vi "Store Packet.vi"(8 "error in (no error)":errorcluster, 9 "last attempt (now)":timestamp, 10 "ControlPacket":refnum<class "ControlPacket.lvclass">, 11 "Subscription in":refnum<class "Subscription.lvclass">) -> (0 "error out":errorcluster, 2 "ControlPacket dup":refnum<class "ControlPacket.lvclass">, 3 "Subscription out":refnum<class "Subscription.lvclass">)   [LabVIEW 2013, in "MQTT Server.lvlib" / "Subscription.lvclass"]
uses:
  Subscription.lvclass
  <vilib>/LabVIEW Open Source Project/MQTT Control Packets/Control Packets/ControlPacket/ControlPacket.lvclass
  Stored Packet -- cluster.ctl
  Subscription.lvclass/Subscription.ctl
  <vilib>/LabVIEW Open Source Project/MQTT Control Packets/Control Packets/ControlPacket/ControlPacket.lvclass/ControlPacket.ctl
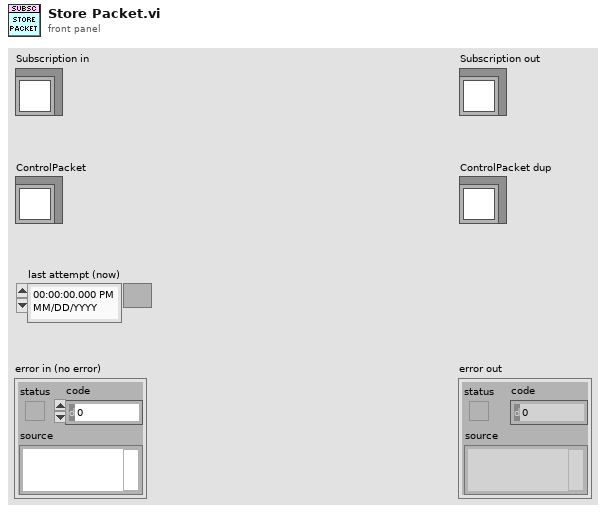
[diagram p1: front panel]
types:
  T1 = typedef "MQTT Server.lvlib/Subscription.lvclass/Stored Packet -- cluster.ctl" = cluster{"Packet Identifier":u16, "ControlPacket":refnum<class "ControlPacket.lvclass">, "last attempt":timestamp}
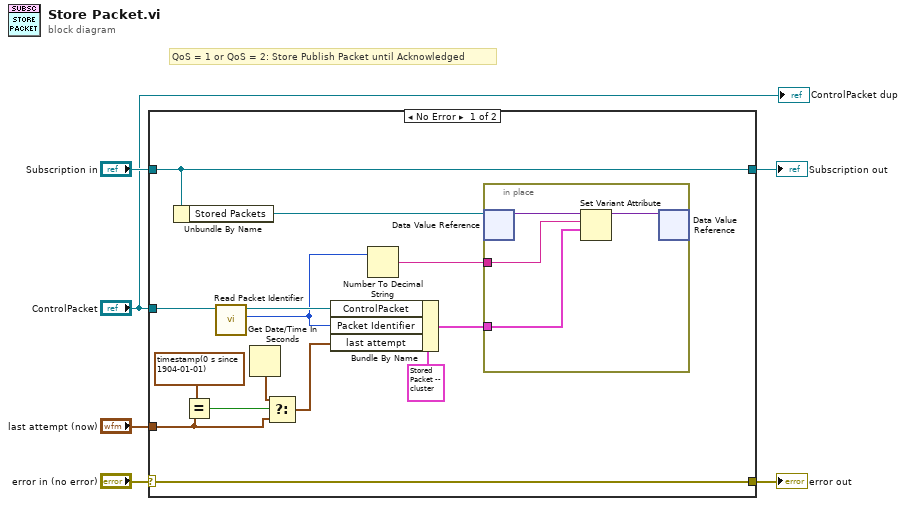
[diagram p0: block diagram]
diagram:
  # "QoS = 1 or QoS = 2: Store Publish Packet until Acknowledged"
  n1 = case shown="No Error" "error in (no error)" {
    selector: "error in (no error)" -> [w20 w26]
    tunnel: [w20 w26] -> w5
    tunnel: [w19 w25] -> w3
    tunnel: "Subscription in" -> [w19 w25]
    tunnel: "ControlPacket" -> [w17 _]
    tunnel: "last attempt (now)" -> [w12 _]
    frame No Error {
      n2 = Unbundle By Name(w19) -> ("Stored Packets"=w18:refnum<data-value>)
      n3 = Equal?(x=timestamp(0 s since 1904-01-01), y=w12) -> (x = y?=w14:bool)
      n4 = call <vilib>:"Read Packet Identifier.vi"("ControlPacket in"=w17) -> ("Packet Identifier"=w9:u16, "ControlPacket out"=w15:refnum<class "ControlPacket.lvclass">)  [unwired: 9 in]
      n5 = Get Date/Time In Seconds() -> (seconds since 1Jan1904=w13:timestamp)
      n6 = Select(t=w13, s=w14, f=w12) -> (s? t:f=w11:timestamp)
      n7 = Bundle By Name(cluster=T1 {"Packet Identifier"=0, "ControlPacket"=refnum, "last attempt"=timestamp(0 s since 1904-01-01)} ("Stored Packet"), "ControlPacket"=w15, "Packet Identifier"=w9, "last attempt"=w11) -> (w10:T1)
      n8 = Number To Decimal String(number=w9) -> (decimal integer string=w8:string)  [unwired: 1 in]
      n9 = in-place {
        in-place-border: w10 -> [w22]
        in-place-border: w8 -> [w21]
        n10 = in-place-dvr #1(w18) -> (w24:variant)  [unwired: 1 out]
        n11 = Set Variant Attribute(Variant=w24, name=w21, value=w22) -> (Variant out=w23:variant)  [unwired: 1 in, 2 out]
        n12 = in-place-dvr #1(w23) -> ()  [unwired: 2 out]
      }
    }
    frame Error {
    }
  }
  "error out" <- w5
  "Subscription out" <- w3
  "ControlPacket dup" <- "ControlPacket"
